vi "Nb Items Per Page--constant.vi"() -> (3 "Nb Items Per Page":i32=50)   [LabVIEW 2020, in "WSsupport.lvlib"]
uses:
  WSsupport.lvlib
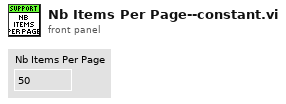
[diagram p1: front panel]
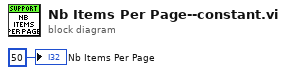
[diagram p0: block diagram]
diagram:
  "Nb Items Per Page" <- 50
